vi "Fetch (Digital Waveform).vi"(7 "Segment Index (0)":i32 format="%.0g", 8 "error in (no error)":errorcluster, 9 "Maximum Time (10000ms)":u32, 10 "Channel (31: POD 1)":i32(ring) items=["POD 1", "POD 2"], 11 "VISA resource name":refnum<visa-resource-name>) -> (0 "error out":errorcluster, 2 "Digital Waveform Graph":digitalwaveform(graph), 3 "VISA resource name out":refnum<visa-resource-name>)   [LabVIEW 2009, in "Agilent 8000 Series.lvlib"]
doc: "Returns the waveform the oscilloscope acquired for the specified channel. The waveform is from an acquisition that you initiate prior to calling this VI.\n\nYou use the Initiate VI to start an acquisition on the channels that you enable with the <B>Configure Channel</B> VI. The oscilloscope acquires waveforms for the enabled channels concurrently. You must call this VI separately for each enabled channel to obtain the waveforms.\n\nYou can call the <B>Read (Digital Waveforms)</B> VI instead of using low level VIs.\n\n<B>Note</B> This VI does not check the instrument status. Typically, you call this VI only in a sequence of calls to other low-level instrument driver VIs. The sequence performs one operation. You use the low-level VIs to optimize one or more aspects of interaction with the instrument."
uses:
  Agilent 8000 Series.lvlib
  <vilib>/Waveform/DWDTOps.llb/DWDT Binary U8 to Digital.vi
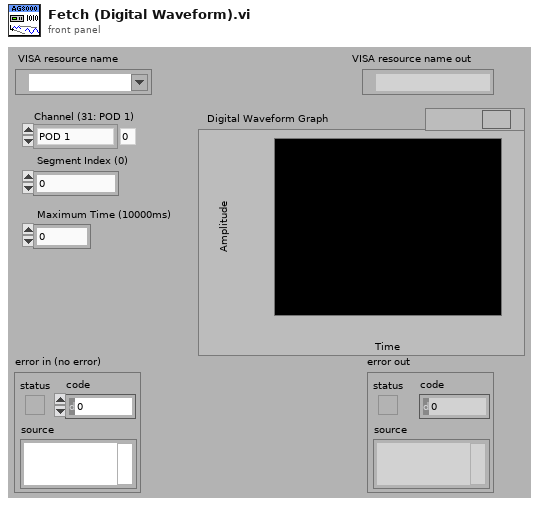
[diagram p1: front panel]
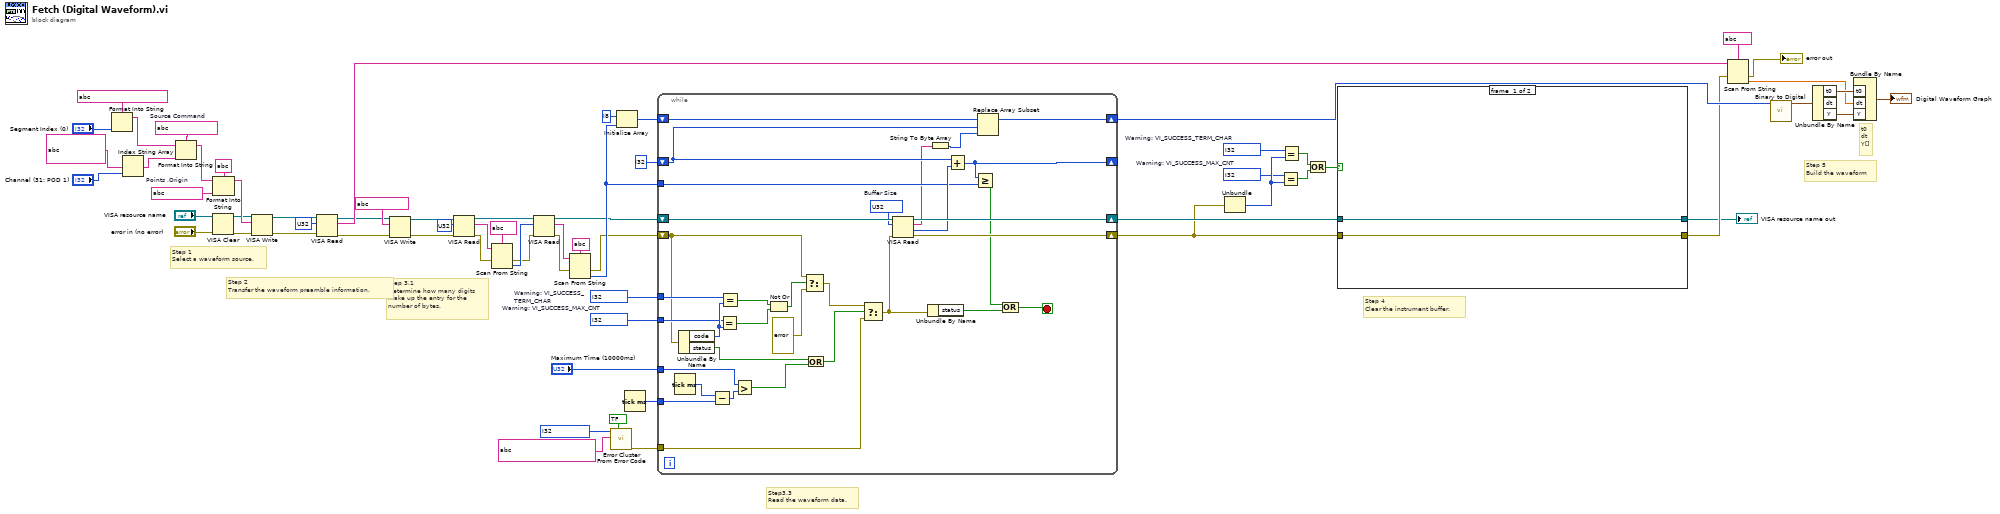
[diagram p0: block diagram]
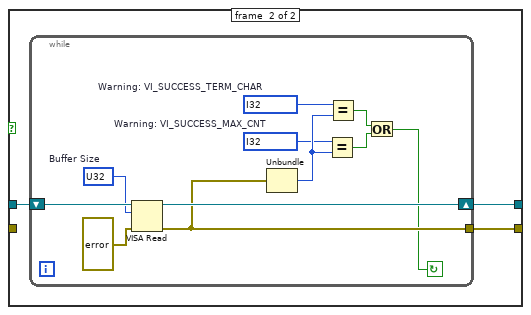
[diagram p2: hidden frame]
diagram:
  w41 = i32 ?  # Warning: VI_SUCCESS_MAX_CNT
  w40 = i32 ?  # Warning: VI_SUCCESS_TERM_CHAR
  w33 = i32 ?  # Warning: VI_SUCCESS_MAX_CNT
  w32 = i32 ?  # Warning: VI_SUCCESS_TERM_CHAR
  w57 = string ?  # Source Command
  w54 = string ?  # Points ,Origin
  # "Step 5    \nBuild the waveform"
  # "Step 4    \nClear the instrument buffer."
  # "Step3.3   \nRead the waveform data."
  # "Step 3.1     \nDetermine how many digits\nmake up the entry for the \nnumber of bytes."
  # "Step 2\nTransfer the waveform preamble information."
  # "Step 1       \nSelect a waveform source."
  # "t0\ndt\nY[]"
  n1 = Format Into String(format string=string ?, "Segment Index (0)") -> (resulting string=w56:string)  [unwired: 2 in, 1 out]
  n2 = Index String Array(1:"Channel (31: POD 1)", 2:string[] ?) -> (0:w6:string)  [unwired: 1 in]
  n3 = Format Into String(format string=w57, initial string=w56, w6) -> (resulting string=w55:string)  [unwired: 1 in, 1 out]
  n4 = VISA Clear(VISA resource name="VISA resource name", error in (no error)="error in (no error)") -> (VISA resource name out=w2:refnum<visa-resource-name>, error out=w1:errorcluster)
  n5 = Format Into String(format string=string ?, initial string=w55, w54) -> (resulting string=w60:string)  [unwired: 1 in, 1 out]
  n6 = VISA Write(VISA resource name=w2, write buffer=w60, error in (no error)=w1) -> (VISA resource name out=w66:refnum<visa-resource-name>, error out=w65:errorcluster)  [unwired: 1 out]
  n7 = VISA Read(VISA resource name=w66, byte count=u32 ?, error in (no error)=w65) -> (VISA resource name out=w9:refnum<visa-resource-name>, read buffer=w62:string, error out=w8:errorcluster)  [unwired: 1 out]
  n8 = VISA Write(VISA resource name=w9, write buffer=string ?, error in (no error)=w8) -> (VISA resource name out=w16:refnum<visa-resource-name>, error out=w15:errorcluster)  [unwired: 1 out]
  n9 = VISA Read(VISA resource name=w16, byte count=u32 ?, error in (no error)=w15) -> (VISA resource name out=w22:refnum<visa-resource-name>, read buffer=w19:string, error out=w18:errorcluster)  [unwired: 1 out]
  n10 = Scan From String(format string=string ?, input string=w19, error in=w18) -> (error out=w21:errorcluster, output 1=w48:i32)  [unwired: 2 in, 2 out]
  n11 = VISA Read(VISA resource name=w22, byte count=w48, error in (no error)=w21) -> (VISA resource name out=w26:refnum<visa-resource-name>, read buffer=w25:string, error out=w23:errorcluster)  [unwired: 1 out]
  n12 = Scan From String(format string=string ?, input string=w25, error in=w23) -> (error out=w27:errorcluster, output 1=w31:i32)  [unwired: 2 in, 2 out]
  n13 = call <vilib>:"Error Cluster From Error Code.vi"("show call chain? (False)"=bool ?, "error message (\"\")"=string ? ("error message (\"\")"), "error code (0)"=i32 ?) -> ("error out"=w39:errorcluster)  [unwired: 6 in]
  n14 = Initialize Array(i8 ? ("element"), w31) -> (w29:i8[])
  n15 = Tick Count (ms)() -> (millisecond timer value=w38:u32)
  n16 = while {
    shift-right: [w94] -> w46
    shift-left: w27 -> [w81]
    shift-right: [w99] -> w47
    shift-left: w26 -> [w98]
    shift-right: [w95] -> w13
    shift-left: w29 -> [w96]
    shift-right: [w91] -> _
    shift-left: i32 ? ("index") -> [w92]
    tunnel: w31 -> [w90]
    tunnel: w32 -> [w83]
    tunnel: w33 -> [w82]
    tunnel: "Maximum Time (10000ms)" -> [w78]
    tunnel: w38 -> [w77]
    tunnel: w39 -> [w72]
    stop <- w69 stop-if-true
    w97 = u32 ?  # Buffer Size
    n17 = Tick Count (ms)() -> (millisecond timer value=w79:u32)
    n18 = Unbundle By Name(w81) -> ("code"=w84:i32, "status"=w76:bool)
    n19 = Subtract(x=w79, y=w77) -> (x-y=w80:u32)
    n20 = Equal?(x=w82, y=w84) -> (x = y?=w87:bool)
    n21 = Equal?(x=w83, y=w84) -> (x = y?=w88:bool)
    n22 = Greater?(x=w78, y=w80) -> (0:w75:bool)
    n23 = Not Or(1:w87, 2:w88) -> (0:w86:bool)
    n24 = Select(t=w81, s=w86, f=errorcluster ? ("error in (no error)")) -> (s? t:f=w74:errorcluster)
    n25 = Or(x=w76, y=w75) -> (x .or. y?=w73:bool)
    n26 = Select(t=w74, s=w73, f=w72) -> (s? t:f=w71:errorcluster)
    n27 = VISA Read(VISA resource name=w98, byte count=w97, error in (no error)=w71) -> (VISA resource name out=w99:refnum<visa-resource-name>, read buffer=w67:string, return count=w93:u32, error out=w94:errorcluster)
    n28 = Unbundle By Name(w71) -> ("status"=w70:bool)
    n29 = String To Byte Array(string=w67) -> (unsigned byte array=w68:u8[])
    n30 = Add(x=w92, y=w93) -> (x+y=w91:u32)
    n31 = Greater Or Equal?(x=w91, y=w90) -> (x >= y?=w89:bool)
    n32 = Replace Array Subset(array=w96, new element=w68, index=w92) -> (w95:i8[])
    n33 = Compound Arithmetic op=OR(w89, w70) -> (w69:bool)
  }
  n34 = Unbundle(w46) -> ("code"=w42:i32)  [unwired: 2 out]
  n35 = Equal?(x=w41, y=w42) -> (x = y?=w44:bool)
  n36 = Equal?(x=w40, y=w42) -> (x = y?=w45:bool)
  n37 = Or(x=w45, y=w44) -> (x .or. y?=w43:bool)
  n38 = case shown="True" w43 {
    tunnel: w47 -> [w101 w104]
    tunnel: w46 -> [w100 _]
    tunnel: [w101 w103] -> w10
    tunnel: [w100 w102] -> w12
    frame #0 {
    }
    frame #1 {
      n39 = while {
        shift-right: [w114] -> w103
        shift-left: w104 -> [w115]
        tunnel: [w107] -> w102
        stop <- w106 continue-if-true
        w109 = i32 ?  # Warning: VI_SUCCESS_MAX_CNT
        w108 = i32 ?  # Warning: VI_SUCCESS_TERM_CHAR
        w113 = u32 ?  # Buffer Size
        n40 = VISA Read(VISA resource name=w115, byte count=w113, error in (no error)=errorcluster ?) -> (VISA resource name out=w114:refnum<visa-resource-name>, error out=w107:errorcluster)  [unwired: 2 out]
        n41 = Unbundle(w107) -> ("code"=w110:i32)  [unwired: 2 out]
        n42 = Equal?(x=w109, y=w110) -> (x = y?=w111:bool)
        n43 = Equal?(x=w108, y=w110) -> (x = y?=w112:bool)
        n44 = Or(x=w112, y=w111) -> (x .or. y?=w106:bool)
      }
    }
  }
  "VISA resource name out" <- w10
  n45 = Scan From String(format string=string ?, input string=w62, error in=w12) -> (error out=→"error out":errorcluster, output 1=w49:dbl)  [unwired: 2 in, 2 out]
  n46 = call-poly <vilib>:"Binary to Digital.vi"("binary array"=w13) -> ("digital waveform"=w50:digitalwaveform)  [unwired: 9 in, 1 out]
  n47 = Unbundle By Name ("Get Waveform Components")(w50) -> ("t0"=w52:timestamp, "Y"=w53:digitaldata)  [unwired: 1 out]
  n48 = Bundle By Name("t0"=w52, "dt"=w49, "Y"=w53) -> (→"Digital Waveform Graph":digitalwaveform)  [unwired: 1 in]
